vi "LINX - Analog IO.vi"() -> ()   [LabVIEW 2020]
uses:
  <vilib>/MakerHub/LINX/Public/Peripherals/Analog/Analog Read 1 Chan.vi
  <vilib>/MakerHub/LINX/Public/Peripherals/Analog/Analog Read N Chans.vi
  <vilib>/MakerHub/LINX/Private/Local IO/LinxAnalogRead.vi
  <vilib>/MakerHub/LINX/Public/Utilities/Check Channel.vi
  <vilib>/MakerHub/LINX/Public/Utilities/Open Serial.vi
  <vilib>/MakerHub/LINX/Public/Peripherals/Analog/Analog Write 1 Chan.vi
  <vilib>/MakerHub/LINX/Private/Utilties/Generate Error.vi
  <vilib>/MakerHub/LINX/LMH-LINX.lvlib
panel:
  in  "iterations per cycle":i32=400
  out "Measured/expected AI":dbl
  out "Loop Rate (Hz)":u32
  out "Waveform Chart":cluster{dbl, "Voltage":dbl}(graph)
  in  "Serial Port":refnum<visa-resource-name>="N/A"
  in  "stop":bool
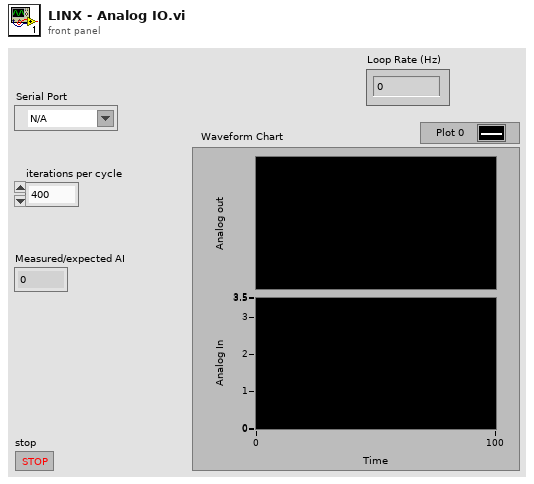
[diagram p1: front panel]
types:
  T1 = typedef "LMH-LINX.lvlib/LINX Ref.ctl" = cluster{"IO":T2, "Interface":T3, "LINX Device Config":T4}
  T2 = typedef "LMH-LINX.lvlib/Platform.ctl" = enum16{"Remote", "Local"}
  T3 = typedef "LMH-LINX.lvlib/Interface.ctl" = enum16{"Serial", "TCP"}
  T4 = typedef "LMH-LINX.lvlib/Device.lvlib/LINX Device Config.ctl" = cluster{"Interface":T3, "COM Port":refnum<visa-resource-name>, "TCP Configuration":T5, "Device Family":u8, "Device ID":u8, "Device Name":string, "TCP Ref":refnum<k5>, "Channels":T6}
  T5 = typedef "LMH-LINX.lvlib/Device.lvlib/TCP Config.ctl" = cluster{"IP Address":string, "Port":u16}
  T6 = typedef "LMH-LINX.lvlib/Channels.ctl" = cluster{"DI":u8[], "DO":u8[], "AI":u8[], "AO":u8[], "PWM":u8[], "QE":u8[], "UART":u8[], "I2C 2":u8[], "SPI":u8[], "CAN":u8[], "Servo":u8[], "AI Ref (V)":dbl, "AI Resolution (Bits)":u8, "AO Ref (V)":dbl, "AO Resolution (Bits)":u8}
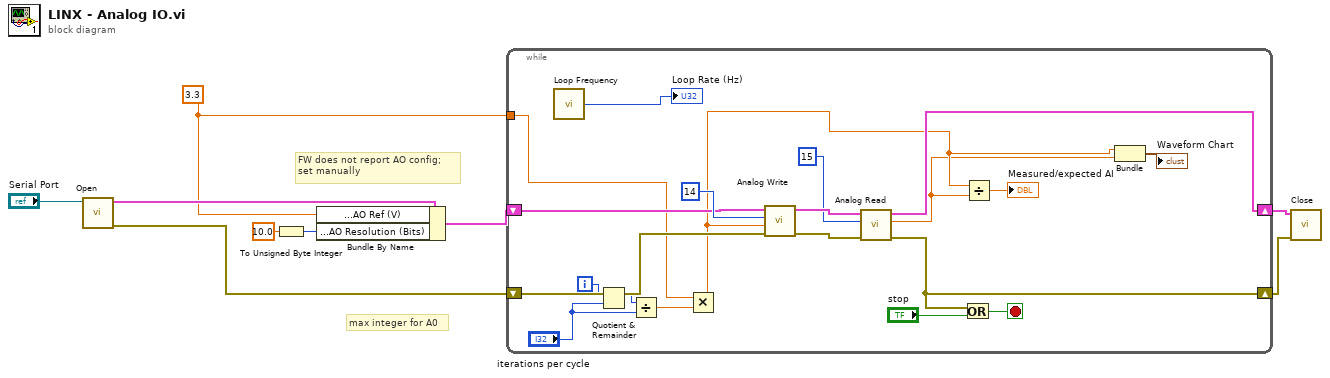
[diagram p0: block diagram]
diagram:
  w2 = 3.3
  # "FW does not report AO config;\nset manually"
  # "max integer for A0"
  n1 = call-poly <vilib>:"Open.vi"("Serial Port"="Serial Port") -> ("Error Out"=w8:errorcluster, "LINX Resource"=w9:T1)  [unwired: 8 in, 1 out]
  n2 = To Unsigned Byte Integer(number=10.0 ("x")) -> (unsigned 8bit integer=w1:u8)
  n3 = Bundle By Name(cluster=w9, "LINX Device Config.Channels.AO Ref (V)"=w2, "LINX Device Config.Channels.AO Resolution (Bits)"=w1) -> (w4:T1)
  n4 = while {
    shift-right: [w20] -> w7
    shift-left: w4 -> [w17]
    shift-right: [w24] -> w6
    shift-left: w8 -> [w29]
    tunnel: w2 -> [w10]
    i -> [w27]
    stop <- w25 stop-if-true
    n5 = call <vilib>:"Loop Frequency.vi"() -> ("Loop Rate (Hz)"=→"Loop Rate (Hz)":u32)
    n6 = Quotient & Remainder(x=w27, y="iterations per cycle") -> (x-y*floor(x/y)=w15:i32)  [unwired: 1 out]
    n7 = Divide(x=w15, y="iterations per cycle") -> (x/y=w14:dbl)
    n8 = Multiply(x=w10, y=w14) -> (x*y=w13:dbl)
    n9 = call-poly <vilib>:"Analog Write.vi"("Error In"=w29, "AO Value"=w13, "AO Channel"=u8 14, "LINX Resource"=w17) -> ("Error Out"=w23:errorcluster, "LINX Resource"=w22:T1)  [unwired: 6 in]
    n10 = call-poly <vilib>:"Analog Read.vi"("Error In"=w23, "Analog Channel"=u8 15, "LINX Resource"=w22) -> ("Error Out"=w24:errorcluster, "Voltage"=w11:dbl, "LINX Resource"=w20:T1)  [unwired: 5 in, 1 out]
    n11 = Or(x=w24, y="stop") -> (x .or. y?=w25:bool)
    n12 = Divide(x=w13, y=w11) -> (x/y=→"Measured/expected AI":dbl)
    n13 = Bundle(w13, "Voltage"=w11) -> (→"Waveform Chart":cluster{dbl, "Voltage":dbl})  [unwired: 1 in]
  }
  n14 = call <vilib>:"Close.vi"("Error In"=w6, "LINX Resource"=w7) -> ()  [unwired: 9 in, 1 out]
